vi "SCM Microphone Test Data Analyzer.vi"() -> ()   [LabVIEW 2013]
panel:
  in  "Image Path":path
  in  "Save PNG":bool
  out "Signal Integrations":dbl[][](graph)
  out "Signal Amplitudes":dbl[][](graph)
  in  "Analyze":bool
  in  "# Channels":i32=24
  in  "stop":bool
  out "Microphone Locations":cluster{"r":dbl, "theta":dbl}[](array[cluster])
  in  "Sample Rate":i32=100000
  in  "Record Position":u32(knob) max=4053 scale=0.0..163.0
  in  "# Records":u32=1 max=163
  in  "Data File":path=path "C:/Users/plane/Desktop/Data/runs-2014_11_21_16_00/runs/2014-11-14/Run_110/NI-Scope_2014-11-14_Run_110.wfm"
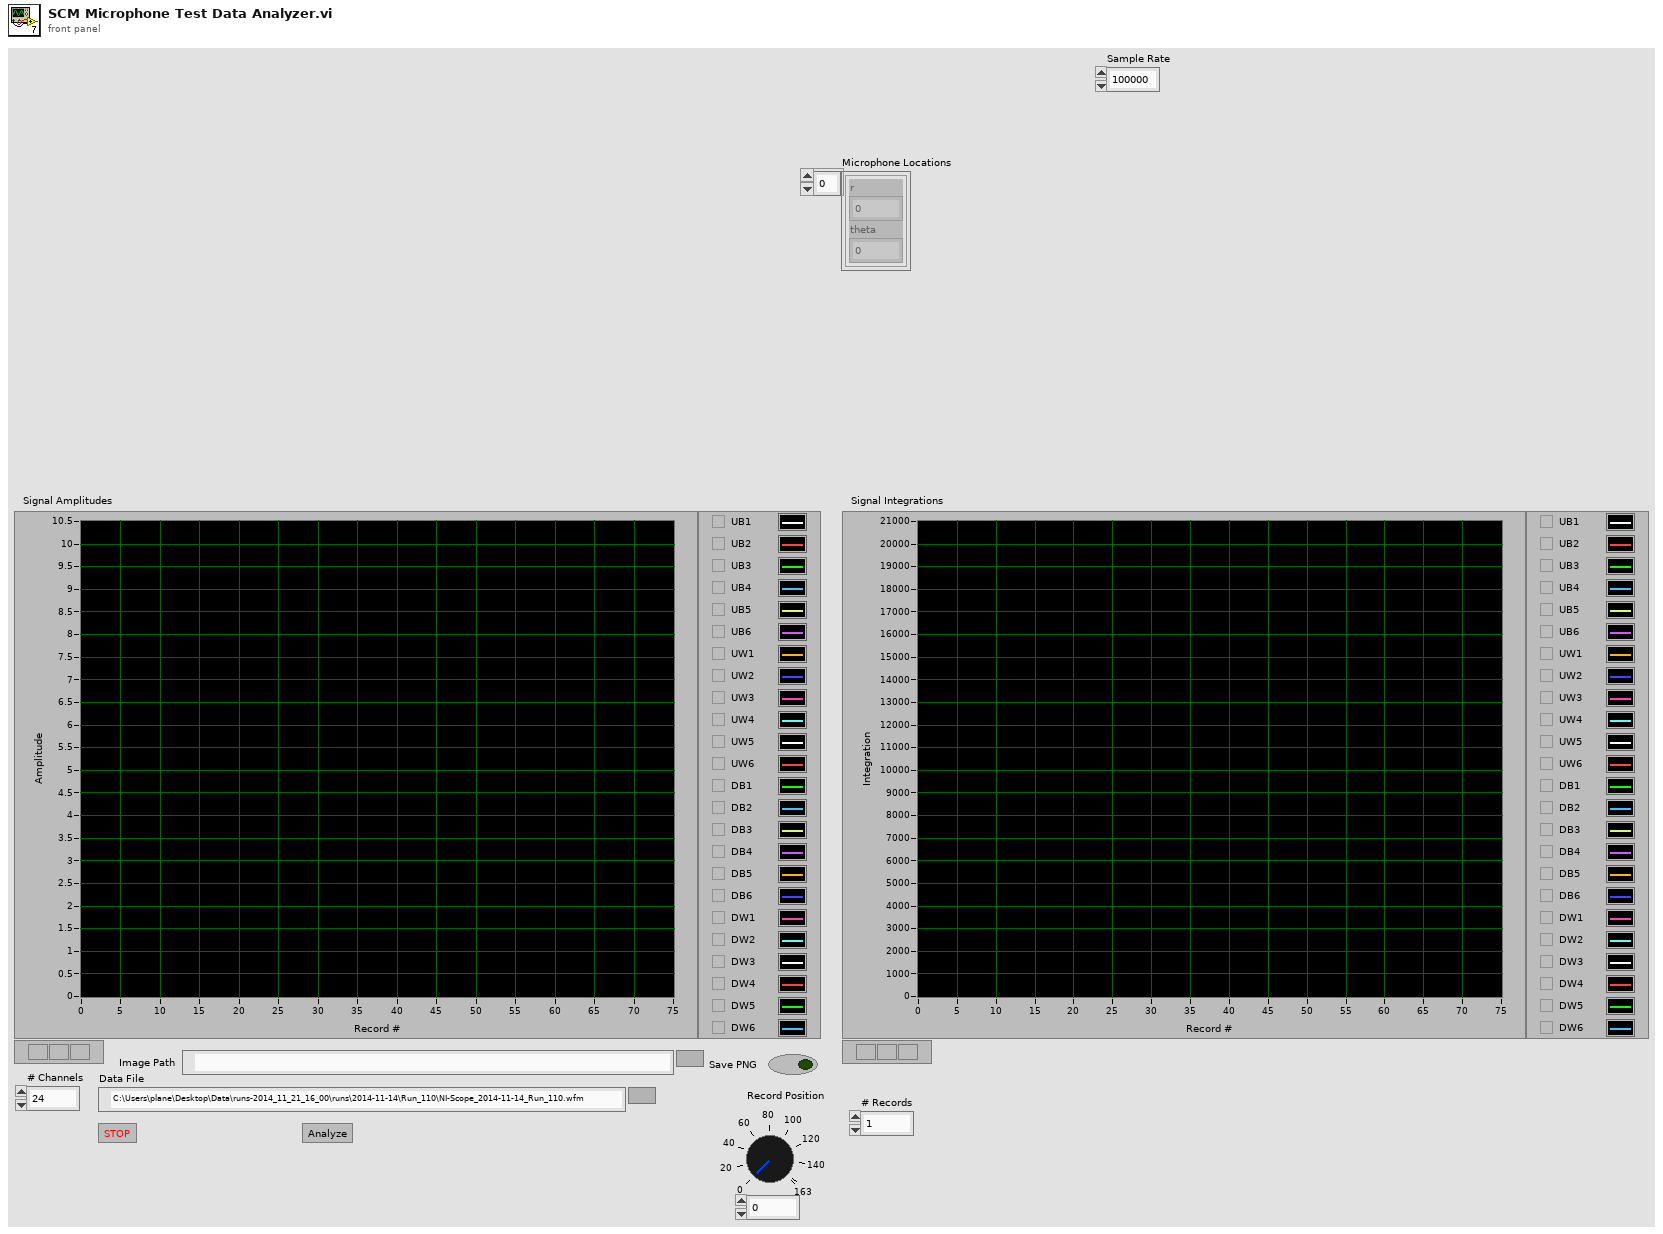
[diagram p1: front panel]
types:
  T1 = enum16{"big-endian, network order", "native, host order", "little-endian"}
  T2 = typedef "imagedata.ctl" = cluster{"image type":i32, "image depth":i32, "image":u8[], "mask":u8[], "colors":u32[], "Rectangle":cluster{"left":i16, "top":i16, "right":i16, "bottom":i16}}
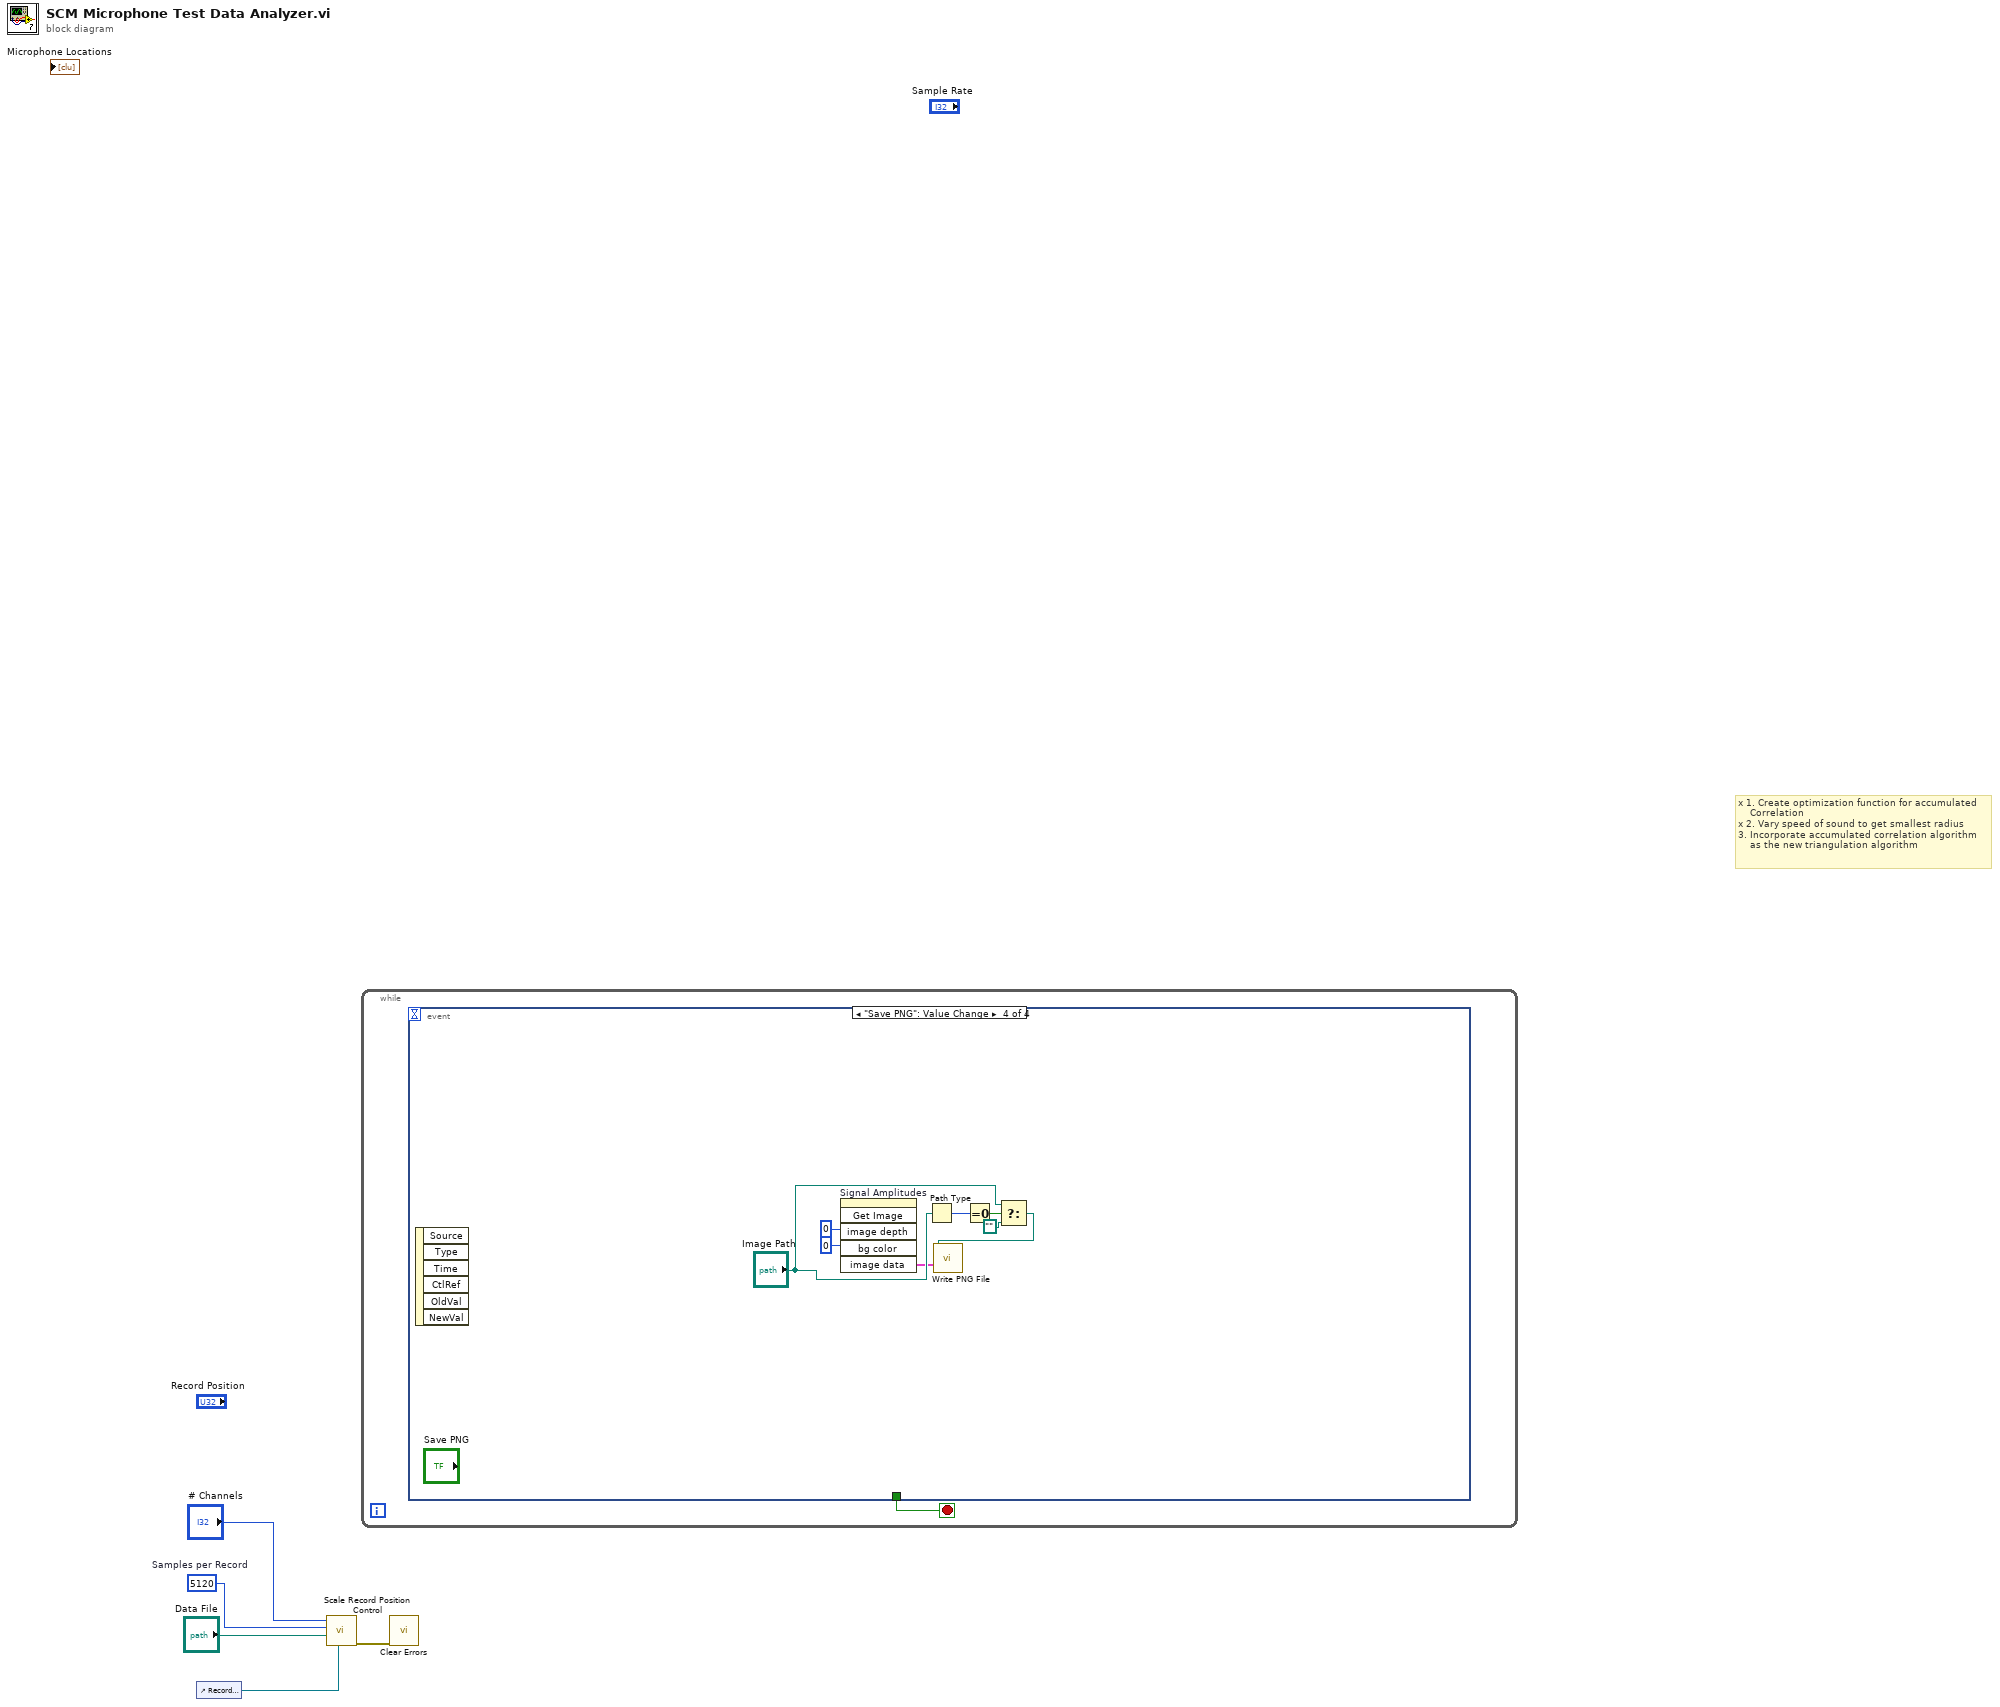
[diagram p0: block diagram]
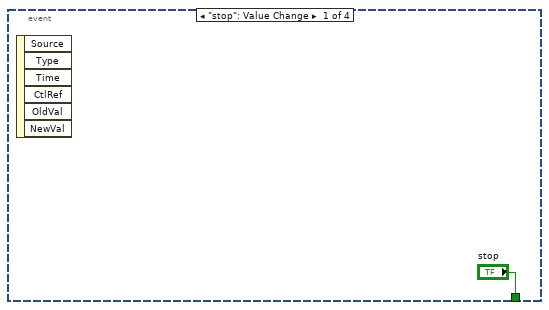
[diagram p2: hidden frame]
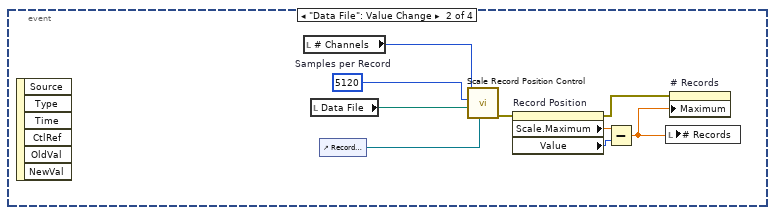
[diagram p3: hidden frame]
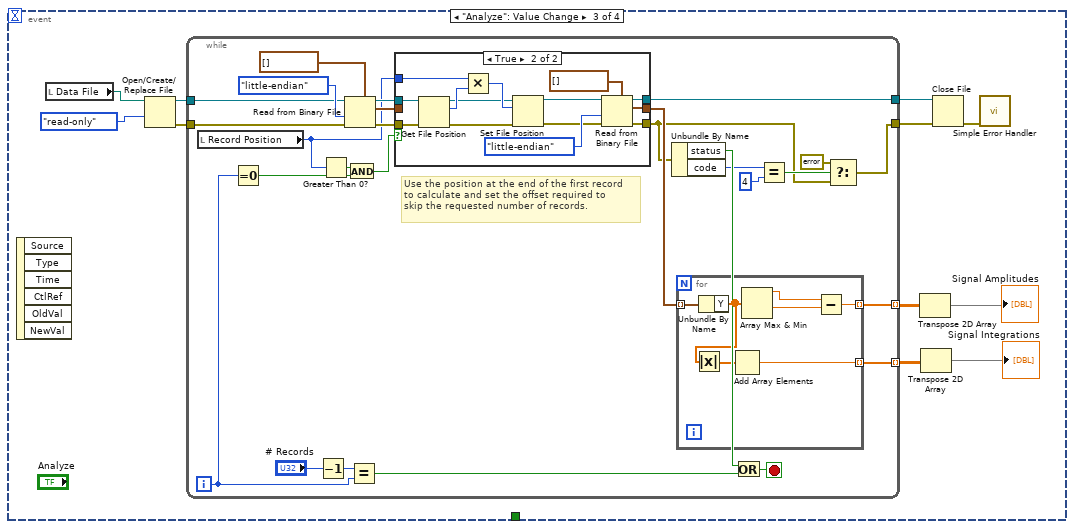
[diagram p4: hidden frame]
diagram:
  w3 = 5120  # Samples per Record
  # "x 1. Create optimization function for accumulated\n    Correlation\nx 2. Vary speed of sound to get smallest radius\n3. Incorporate accumulated correlation algorithm\n    as the new triangulation algorithm"
  n1 = control-ref of="Record Position"() -> (w2:refnum<vi>)
  n2 = call "Scale Record Position Control.vi"("Record Pos. Ref."=w2, "Data File Path"="Data File", "Samples per Record"=w3, "# Channels"="# Channels") -> ("error out"=w1:errorcluster)  [unwired: 7 in]
  n3 = while {
    stop <- w6 stop-if-true
    n4 = event shown="[3] \"Save PNG\": Value Change" {
      selector: _ -> [_ _ _ _]
      dyn-events: _ -> [_ _ _ _]
      timeout: _ -> [_ _ _ _]
      tunnel: ["stop" _ _ _] -> w6
      event "stop": Value Change {
        n5 = event-data() -> ()  [unwired: 1 in, 6 out]
      }
      event "Data File": Value Change {
        w15 = 5120  # Samples per Record
        n6 = event-data() -> ()  [unwired: 1 in, 6 out]
        n7 = local read "# Channels"() -> (w14:i32)
        n8 = local read "Data File"() -> (w16:path)
        n9 = control-ref of="Record Position"() -> (w13:refnum<vi>)
        n10 = call "Scale Record Position Control.vi"("Record Pos. Ref."=w13, "Data File Path"=w16, "Samples per Record"=w15, "# Channels"=w14) -> ("error out"=w12:errorcluster)  [unwired: 7 in]
        n11 = property on="Record Position" class="Knob (strict)"(error in=w12) -> (error out=w9:errorcluster, "Scale.Maximum"=w11:dbl, "Value"=w10:u32)  [unwired: 1 in, 1 out]
        n12 = Subtract(x=w11, y=w10) -> (x-y=w8:dbl)
        n13 = local write "# Records"(w8) -> ()
        n14 = property on="# Records" class="DigNum (strict)"(error in=w9, "Maximum"=w8) -> ()  [unwired: 1 in, 2 out]
      }
      event "Analyze": Value Change {
        n15 = event-data() -> ()  [unwired: 1 in, 6 out]
        n16 = local read "Data File"() -> (w27:path)
        n17 = Open/Create/Replace File(file path (use dialog)=w27, access (0:read/write)=enum16{"read/write", "read-only", "write-only"}."read-only") -> (refnum out=w23:refnum<file>, error out=w24:errorcluster)  [unwired: 4 in, 1 out]
        n18 = while {
          tunnel: w23 -> [w49]
          tunnel: w24 -> [w48]
          tunnel: [w40] -> w25
          tunnel: [w29] -> w21
          tunnel: [w30] -> w19 mode=indexing
          tunnel: [w28] -> w18 mode=indexing
          i -> [w47]
          stop <- w54 stop-if-true
          # "Use the position at the end of the first record\nto calculate and set the offset required to\nskip the requested number of records."
          n19 = local read "Record Position"() -> (w38:u32)
          n20 = Equal To 0?(x=w47) -> (x = 0?=w42:bool)
          n21 = Decrement(x="# Records") -> (x-1=w39:u32)
          n22 = Greater Than 0?(x=w38) -> (x > 0?=w43:bool)
          n23 = Read from Binary File(5:waveform(dbl)[] [] ("Difference"), 8:w48, 9:T1."little-endian" ("byte order (0:big-endian, network order)"), 11:w49) -> (0:w45:errorcluster, 2:w41:waveform(dbl)[], 3:w46:refnum<file>)  [unwired: 2 in, 1 out]
          n24 = And(x=w43, y=w42) -> (x .and. y?=w44:bool)
          n25 = Equal?(x=w39, y=w47) -> (x = y?=w52:bool)
          n26 = case shown="True" w44 {
            tunnel: w46 -> [w63 w78]
            tunnel: w45 -> [w62 w77]
            tunnel: w38 -> [_ w75]
            tunnel: w41 -> [w64 _]
            tunnel: [w64 w67] -> w36
            tunnel: [w62 w66] -> w31
            tunnel: [w63 w65] -> w40
            frame False {
            }
            frame True {
              n27 = Get File Position(4:w77, 7:w78) -> (0:w73:errorcluster, 2:w76:i64, 3:w72:refnum<file>)
              n28 = Multiply(x=w75, y=w76) -> (x*y=w74:i64)
              n29 = Set File Position(offset (in bytes) (0)=w74, refnum=w72, error in=w73) -> (refnum out=w70:refnum<file>, error out=w68:errorcluster)  [unwired: 1 in]
              n30 = Read from Binary File(5:waveform(dbl)[] [] ("Difference"), 8:w68, 9:T1."little-endian" ("byte order (0:big-endian, network order)"), 11:w70) -> (0:w66:errorcluster, 2:w67:waveform(dbl)[], 3:w65:refnum<file>)  [unwired: 2 in, 1 out]
            }
          }
          n31 = Unbundle By Name(w31) -> ("status"=w53:bool, "code"=w32:i32)
          n32 = for {
            tunnel: w36 -> [w61] mode=indexing
            tunnel: [w58] -> w30 mode=indexing
            tunnel: [w55] -> w28 mode=indexing
            n33 = Unbundle By Name(w61) -> ("Y"=w57:dbl[])
            n34 = Absolute Value(x=w57) -> (abs(x)=w56:dbl[])
            n35 = Add Array Elements(numeric array=w56) -> (sum=w55:dbl)
            n36 = Array Max & Min(array=w57) -> (max value=w60:dbl, min value=w59:dbl)  [unwired: 2 out]
            n37 = Subtract(x=w60, y=w59) -> (x-y=w58:dbl)
          }
          n38 = Or(x=w53, y=w52) -> (x .or. y?=w54:bool)
          n39 = Equal?(x=w32, y=4 ("code")) -> (x = y?=w33:bool)
          n40 = Select(t=errorcluster {"status"=FALSE, "code"=0, "source"=""}, s=w33, f=w31) -> (s? t:f=w29:errorcluster)
        }
        n41 = Transpose 2D Array(2D array=w19) -> (transposed array=→"Signal Amplitudes":dbl[][])
        n42 = Transpose 2D Array(2D array=w18) -> (transposed array=→"Signal Integrations":dbl[][])
        n43 = Close File(refnum=w25, error in=w21) -> (error out=w26:errorcluster)  [unwired: 1 out]
        n44 = call <vilib>:"Simple Error Handler.vi"("error in (no error)"=w26) -> ()  [unwired: 4 in, 5 out]
      }
      event "Save PNG": Value Change {
        n45 = event-data() -> ()  [unwired: 1 in, 6 out]
        n46 = invoke on="Signal Amplitudes" class="WFGraph (strict)" method="Get Image"("image depth"=0 ("Image Depth"), "bg color"=u32 0 ("Background Color")) -> ("image data"=w83:T2)  [unwired: 4 in, 5 out]
        n47 = Path Type(1:"Image Path") -> (0:w82:i16)
        n48 = Equal To 0?(x=w82) -> (x = 0?=w81:bool)
        n49 = Select(t="Image Path", s=w81, f=path "") -> (s? t:f=w80:path)
        n50 = call <vilib>:"Write PNG File.vi"("image data"=w83, "path to PNG file"=w80) -> ()  [unwired: 8 in, 2 out]
      }
    }
  }
  n51 = call <vilib>:"Clear Errors.vi"("error in (no error)"=w1) -> ()  [unwired: 6 in, 1 out]
